vi "EnumCalculos.vi"() -> ()   [LabVIEW 2020]
panel:
  in  "Enum":T1(ring)
  in  "Valor 2":dbl
  in  "Valor 1":dbl
  out "Resultado":dbl
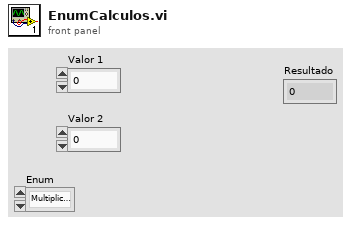
[diagram p1: front panel]
types:
  T1 = enum16{"Multiplicacion", "Divicio", "Resta", "Suma"}
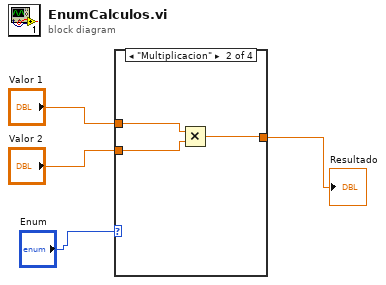
[diagram p0: block diagram]
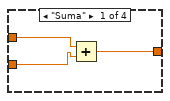
[diagram p2: hidden frame]
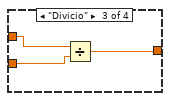
[diagram p3: hidden frame]
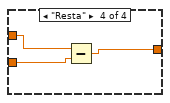
[diagram p4: hidden frame]
diagram:
  n1 = case shown="\"Multiplicacion\"" "Enum" {
    tunnel: "Valor 1" -> [w7 w10 w13 w16]
    tunnel: "Valor 2" -> [w6 w9 w12 w15]
    tunnel: [w5 w8 w11 w14] -> w2
    frame "Suma" {
      n2 = Add(x=w7, y=w6) -> (x+y=w5:dbl)
    }
    frame "Multiplicacion" {
      n3 = Multiply(x=w10, y=w9) -> (x*y=w8:dbl)
    }
    frame "Divicio" {
      n4 = Divide(x=w13, y=w12) -> (x/y=w11:dbl)
    }
    frame "Resta" {
      n5 = Subtract(x=w16, y=w15) -> (x-y=w14:dbl)
    }
  }
  "Resultado" <- w2
